vi "Load_from_Project.vi"(8 "error in (no error)":errorcluster, 9 "index":string, 10 "buildObject":T1, 11 "IB_RegData_String in":refnum<class "IB_RegData_String.lvclass">) -> (0 "error out":errorcluster, 1 "index out":string, 2 "buildObject out":T1, 3 "IB_RegData_String out":refnum<class "IB_RegData_String.lvclass">)   [LabVIEW 2020, in "IB_RegData_String.lvclass"]
uses:
  <vilib>/AppBuilder/IB_Classes/RegData/RegData_String/IB_RegData_String.lvclass
  <vilib>/AppBuilder/IB_Classes/RegData/RegData_String/IB_RegData_String.lvclass/IB_RegData_String.ctl
  <vilib>/AppBuilder/IB_Classes/RegData/IB_RegData.lvclass
  <vilib>/AppBuilder/IB_RW_Project/IB_RW_Project_PropBag_Action.ctl
  <resource>/Framework/Providers/API/ItemRef.ctl
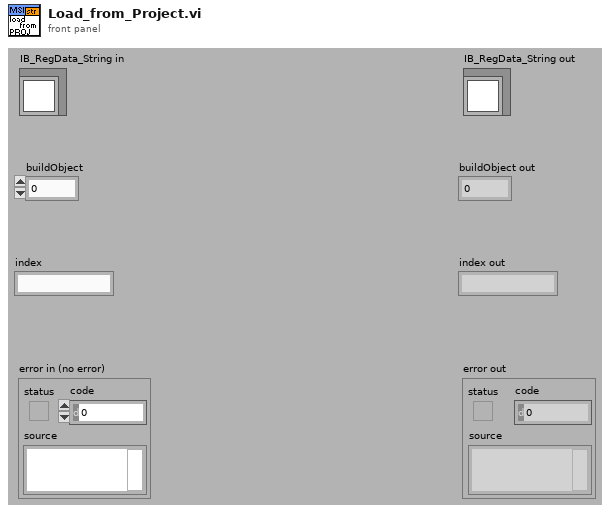
[diagram p1: front panel]
types:
  T1 = typedef "ItemRef.ctl" = u64
  T2 = typedef "IB_RW_Project_PropBag_Action.ctl" = enum16{"read", "write", "clear", "readPrevious", "writePrevious", "clearPrevious"}
  T3 = typedef "IB_RW_Project_RegData_String_Data.ctl" = cluster{"string":string}
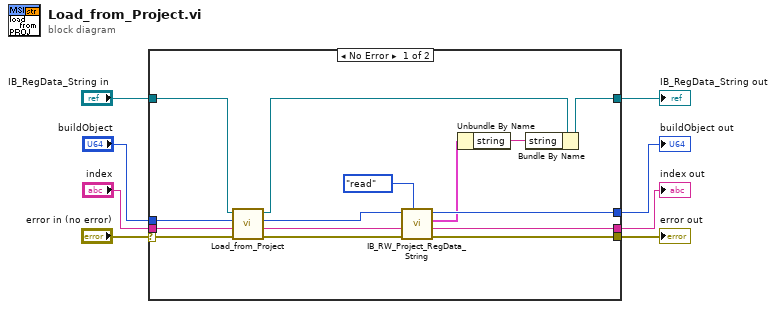
[diagram p0: block diagram]
diagram:
  n1 = case shown="No Error" "error in (no error)" {
    selector: "error in (no error)" -> [w20 w27]
    tunnel: [w13 w27] -> w8
    tunnel: [w18 w24] -> w7
    tunnel: [w16 w25] -> w6
    tunnel: [w11 w26] -> w5
    tunnel: "index" -> [w23 w24]
    tunnel: "buildObject" -> [w22 w25]
    tunnel: "IB_RegData_String in" -> [w21 w26]
    frame No Error {
      n2 = call-parent "Load_from_Project.vi"("error in (no error)"=w20, "index"=w23, "buildObject"=w22, "IB_RegData in"=w21) -> ("error out"=w14:errorcluster, "index out"=w19:string, "buildObject out"=w17:T1, "IB_RegData out"=w12:refnum<class "IB_RegData_String.lvclass">)  [unwired: 4 in]
      n3 = call <vilib>:"IB_RW_Project_RegData_String.vi"("action"=IB_RW_Project_PropBag_Action."read", "error in (no error)"=w14, "index in"=w19, "buildObject"=w17) -> ("error out"=w13:errorcluster, "index out"=w18:string, "RegData"=w10:T3, "buildObject out"=w16:T1)  [unwired: 4 in]
      n4 = Unbundle By Name(w10) -> ("string"=w9:string)
      n5 = Bundle By Name(cluster=w12, "string"=w9) -> (w11:refnum<class "IB_RegData_String.lvclass">)
    }
    frame Error {
    }
  }
  "error out" <- w8
  "IB_RegData_String out" <- w5
  "buildObject out" <- w6
  "index out" <- w7
